vi "TestVI_PowerMeter.vi"() -> ()   [LabVIEW 2018]
uses:
  <vilib>/express/express shared/transition.llb/Dynamic To Waveform Array.vi
  <vilib>/express/express signal manip/GetorSetDDTAttributes/Set DDT Attributes/SetT0.vi
  <vilib>/express/express shared/transition.llb/Waveform Array To Dynamic.vi
  <vilib>/express/express signal manip/GetorSetDDTAttributes/Set DDT Attributes/Set DDT Properties.xnode
panel:
  in  "Save TDMS?":bool
  in  "Projects":string[](array[string])
  in  "Independent?":bool=TRUE
  in  "File Close Action":enum16{"Prompt", "Keep", "Archive", "Trash"}(ring)
  out "VI name":string="TestVI_PowerMeter"
  out "file path":path=path "C:/Users/aspit/Git/MHDLab/Test Data/2018-06-02/H2TC/Temp Dependence/TestVI_PowerMeter_200C.tdms"
  in  "File Information":T1={"Project"=0, "SubFolder"="Temp Dependence", "Filename (Meas. Description)"="200C", "Measurement number"=0} {"Project" items=["H2DT", "VaporTubes", "MaterialsTesting", "ThermalCond", "SeedFeeder", "Rando"]}
  out "tdms error":errorcluster
  out "tdms file":refnum<k34>
  out "output cluster":cluster{"Sine with Uniform Noise":dynamicdata}={"Sine with Uniform Noise"=[{"t0"=timestamp(3610818365.554086 s since 1904-01-01), "dt"=0.001, "Y"=[0.4178071453566156], "attributes"=variant("NI_ChannelName"=variant(string "Sine with Uniform Noise"), "NI_ExpIsRelativeTime"=variant(bool FALSE), "NI_ExpStartTimeStamp"=variant(timestamp timestamp(3610818355.8010864 s since 1904-01-01)), "NI_ExpTimeStamp"=variant(timestamp timestamp(3610818365.554086 s since 1904-01-01)), "NI_ExpXDimension"=variant(string "t"))}]}
  out "Sine with Uniform Noise":dbl=0.4178071453566156
  in  "stop":bool
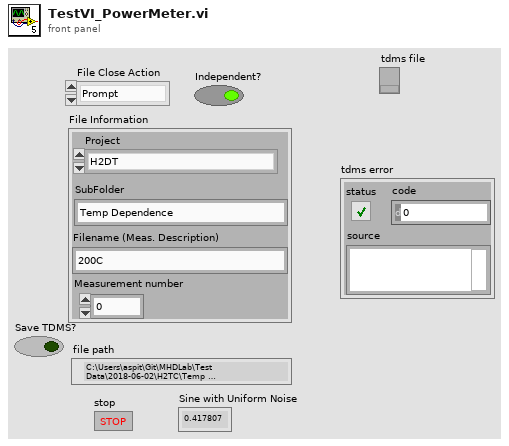
[diagram p1: front panel]
types:
  T1 = cluster{"Project":u16, "SubFolder":string, "Filename (Meas. Description)":string, "Measurement number":i32}
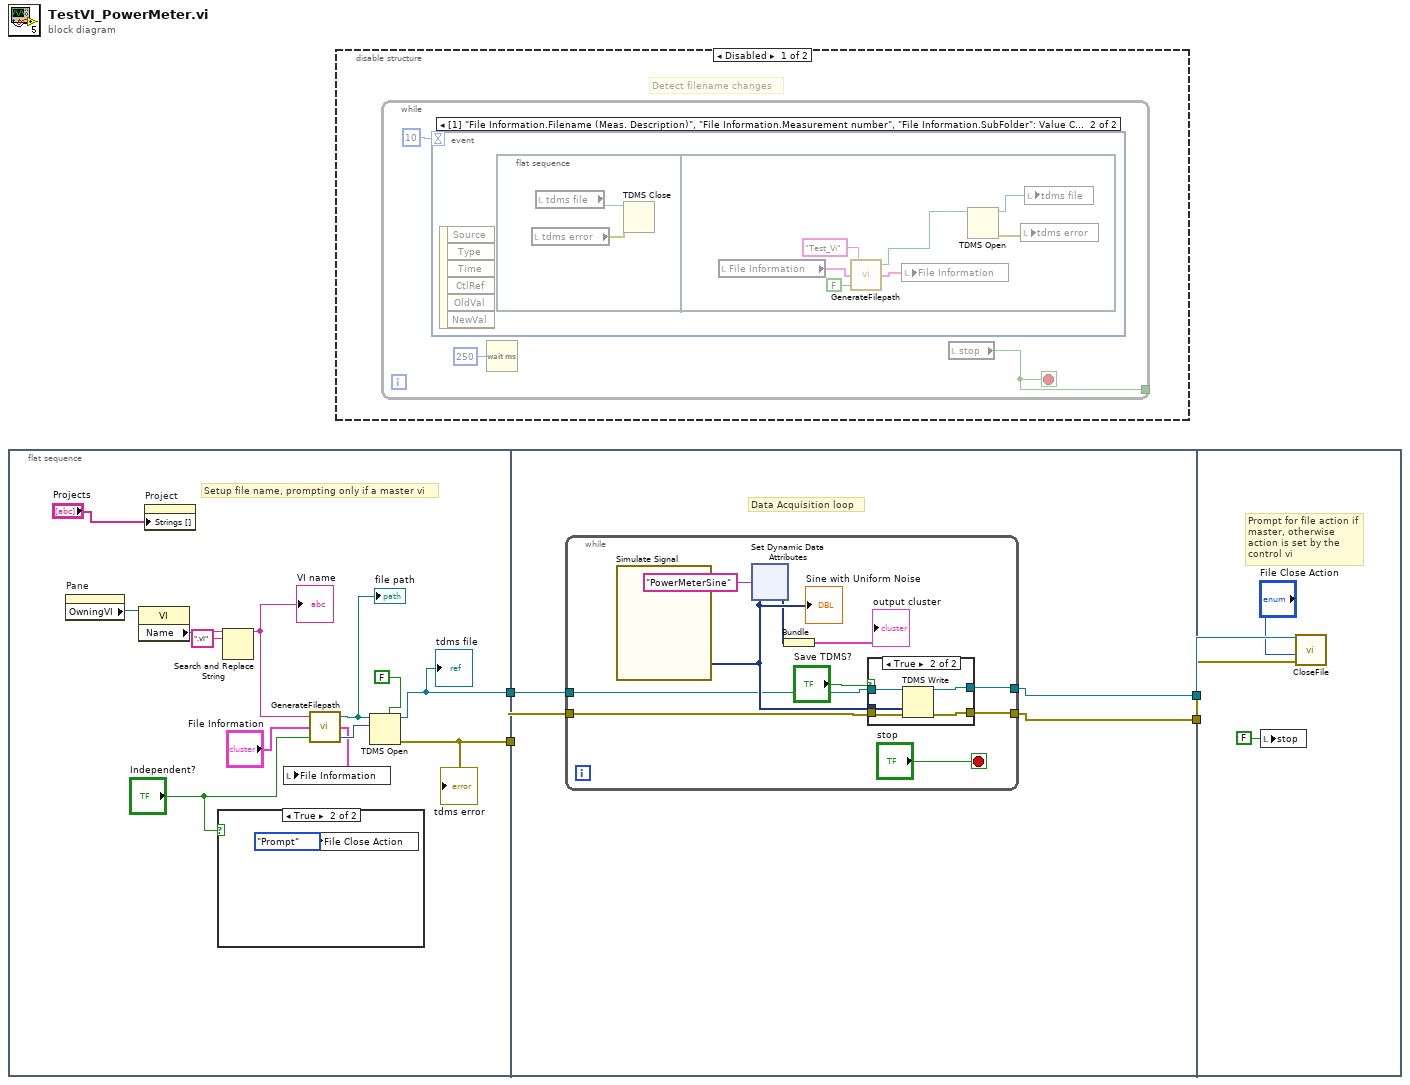
[diagram p0: block diagram]
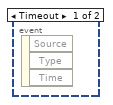
[diagram p4: hidden frame]
diagram:
  n1 = flat-sequence {
    tunnel: [w10] -> w4
    tunnel: [w9] -> w3
    tunnel: w4 -> [w22]
    tunnel: w3 -> [w21]
    tunnel: [w20] -> w2
    tunnel: [w19] -> w1
    tunnel: w2 -> [w56]
    tunnel: w1 -> [w57]
    frame #0 {
      # "Setup file name, prompting only if a master vi"
      n2 = property on="Pane" class="Pane"() -> ("OwningVI"=w16:refnum<vi>)  [unwired: 2 in, 2 out]
      n3 = property class="VI"(reference=w16) -> ("Name"=w17:string)  [unwired: 1 in, 2 out]
      n4 = property on="Project" class="Ring (strict)"("Strings []"="Projects") -> ()  [unwired: 2 in, 2 out]
      n5 = case shown="True" "Independent?" {
        frame False {
        }
        frame True {
          n6 = local write "File Close Action"(enum16{"Prompt", "Keep", "Archive", "Trash"}."Prompt" ("File Close Action")) -> ()
        }
      }
      n7 = Search and Replace String(input string=w17, search string=".vi") -> (result string=w8:string)  [unwired: 6 in, 3 out]
      "VI name" <- w8
      n8 = call "GenerateFilepath.vi"("Check for file?"="Independent?", "File Information"="File Information", "Instrument"=w8) -> ("File Action"=w14:i32, "File Information Out"=w13:T1, "File Path Out"=w7:path)
      "file path" <- w7
      n9 = local write "File Information"(w13) -> ()
      n10 = TDMS Open(5:FALSE ("create index file? (T)"), 10:w14, 11:w7) -> (0:w10:errorcluster, 3:w9:refnum<k34>)  [unwired: 4 in]
      "tdms file" <- w9
      "tdms error" <- w10
    }
    frame #1 {
      # "Data Acquisition loop"
      n11 = while {
        tunnel: [w29] -> w19
        tunnel: [w28] -> w20
        tunnel: w22 -> [w27]
        tunnel: w21 -> [w26]
        stop <- "stop" stop-if-true
        n12 = call "Simulate Signal"() -> ("Sine with Uniform Noise"=w30:dynamicdata)  [unwired: 14 in, 1 out]
        "Sine with Uniform Noise" <- w30
        n13 = xnode "Set Dynamic Data Attributes"("Signals In"=w30, "Signal Name"="PowerMeterSine") -> ("Signals Out"=w24:dynamicdata)  [unwired: 2 in, 1 out]
        n14 = Bundle("Signals Out"=w24) -> (→"output cluster":cluster{"Signals Out":dynamicdata})  [unwired: 1 in]
        n15 = case shown="True" "Save TDMS?" {
          tunnel: w30 -> [_ w53]
          tunnel: [w48 w52] -> w29
          tunnel: [w47 w51] -> w28
          tunnel: w27 -> [w47 w50]
          tunnel: w26 -> [w48 w49]
          frame False {
          }
          frame True {
            n16 = TDMS Write(0:w49, 9:w53, 11:w50) -> (4:w52:refnum<k34>, 15:w51:errorcluster)  [unwired: 3 in, 2 out]
          }
        }
      }
    }
    frame #2 {
      # "Prompt for file action if master, otherwise action is set by the control vi"
      n17 = local write "stop"(FALSE ("stop")) -> ()
      n18 = call "CloseFile.vi"("error in (no error)"=w56, "Action"="File Close Action", "Refnum in"=w57) -> ()  [unwired: 8 in, 1 out]
    }
  }
  n19 = disable-structure shown="Disabled" {
    frame Disabled {
      # "Detect filename changes"
      n20 = while {
        tunnel: [w58] -> _
        stop <- w58 stop-if-true
        n21 = event shown="[1] \"File Information.Filename (Meas. Description)\", \"File Information.Measurement number\", \"File Information.SubFolder\": Value Change" {
          selector: _ -> [_ _]
          dyn-events: _ -> [_ _]
          timeout: 10 -> [_ _]
          event Timeout {
            n22 = event-data() -> ()  [unwired: 1 in, 3 out]
          }
          event "File Information.Filename (Meas. Description)", "File Information.Measurement number", "File Information.SubFolder": Value Change {
            n23 = event-data() -> ()  [unwired: 1 in, 6 out]
            n24 = flat-sequence {
              frame #0 {
                n25 = local read "tdms error"() -> (w62:errorcluster)
                n26 = local read "tdms file"() -> (w61:refnum<k34>)
                n27 = TDMS Close(8:w62, 11:w61) -> ()  [unwired: 2 out]
              }
              frame #1 {
                n28 = local read "File Information"() -> (w67:T1)
                n29 = call "GenerateFilepath.vi"("Check for file?"=FALSE, "File Information"=w67, "Instrument"="Test_Vi") -> ("File Information Out"=w69:T1, "File Path Out"=w66:path)  [unwired: 1 out]
                n30 = local write "File Information"(w69) -> ()
                n31 = TDMS Open(11:w66) -> (0:w64:errorcluster, 3:w65:refnum<k34>)  [unwired: 6 in]
                n32 = local write "tdms error"(w64) -> ()
                n33 = local write "tdms file"(w65) -> ()
              }
            }
          }
        }
        n34 = Wait (ms)(milliseconds to wait=u32 250) -> ()  [unwired: 1 out]
        n35 = local read "stop"() -> (w58:bool)
      }
    }
    frame Enabled {
    }
  }
